vi "oa_SCL Draw Grid.vi"(8 "grid cosmetics":T1={"line color"=39168, "text color"=65280, "tick length"=3, "crossing axes"=FALSE, "visible grid?"=TRUE}, 9 "y scale specs":cluster{"coordinate":i16, "label":string}[](array[cluster]), 10 "x scale specs":cluster{"coordinate":i16, "label":string}[](array[cluster]), 11 "picture":picture) -> (3 "new picture":picture)   [LabVIEW 2017]
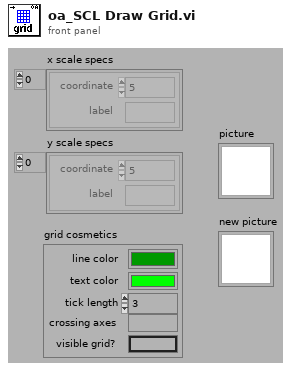
[diagram p1: front panel]
types:
  T1 = cluster{"line color":u32, "text color":u32, "tick length":i16, "crossing axes":bool, "visible grid?":bool}
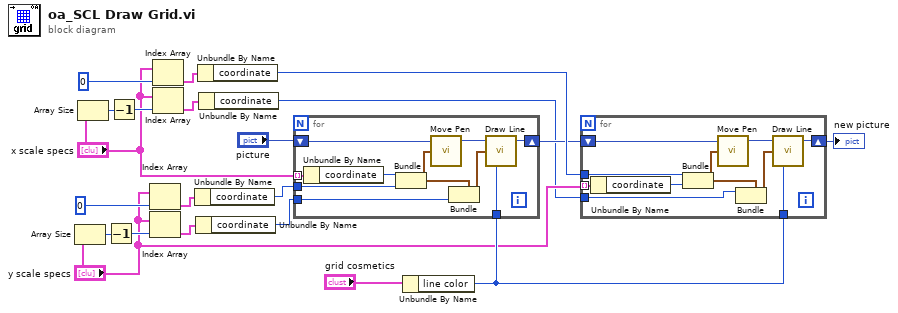
[diagram p0: block diagram]
diagram:
  n1 = Array Size(array="y scale specs") -> (size(s)=w18:i32)
  n2 = Array Size(array="x scale specs") -> (size(s)=w5:i32)
  n3 = Decrement(x=w18) -> (x-1=w19:i32)
  n4 = Decrement(x=w5) -> (x-1=w4:i32)
  n5 = Index Array(array="y scale specs", index=0) -> (element=w16:cluster{"coordinate":i16, "label":string})
  n6 = Index Array(array="y scale specs", index=w19) -> (element=w15:cluster{"coordinate":i16, "label":string})
  n7 = Index Array(array="x scale specs", index=0) -> (element=w7:cluster{"coordinate":i16, "label":string})
  n8 = Index Array(array="x scale specs", index=w4) -> (element=w8:cluster{"coordinate":i16, "label":string})
  n9 = Unbundle By Name(w16) -> ("coordinate"=w14:i16)
  n10 = Unbundle By Name(w15) -> ("coordinate"=w13:i16)
  n11 = Unbundle By Name(w7) -> ("coordinate"=w21:i16)
  n12 = Unbundle By Name(w8) -> ("coordinate"=w1:i16)
  n13 = Unbundle By Name("grid cosmetics") -> ("line color"=w20:u32)
  n14 = for {
    tunnel: "x scale specs" -> [w28] mode=indexing
    tunnel: w14 -> [w26]
    tunnel: w13 -> [w24]
    shift-right: [w31] -> w10
    shift-left: "picture" -> [w29]
    tunnel: w20 -> [w22]
    n15 = Unbundle By Name(w28) -> ("coordinate"=w27:i16)
    n16 = Bundle("coordinate"=w27, "coordinate"=w26) -> (w25:cluster{"coordinate":i16, "coordinate":i16})  [unwired: 1 in]
    n17 = call <vilib>:"Move Pen.vi"("new position"=w25, "picture"=w29) -> ("new picture"=w30:picture)  [unwired: 3 in]
    n18 = Bundle(cluster=w25, "coordinate"=w24) -> (w23:cluster{"coordinate":i16, "coordinate":i16})  [unwired: 1 in]
    n19 = call <vilib>:"Draw Line.vi"("picture"=w30, "end point"=w23, "color(black)"=w22) -> ("new picture"=w31:picture)  [unwired: 6 in]
  }
  n20 = for {
    tunnel: "y scale specs" -> [w38] mode=indexing
    tunnel: w21 -> [w33]
    shift-right: [w41] -> w2
    shift-left: w10 -> [w39]
    tunnel: w20 -> [w35]
    tunnel: w1 -> [w32]
    n21 = Unbundle By Name(w38) -> ("coordinate"=w34:i16)
    n22 = Bundle("coordinate"=w33, "coordinate"=w34) -> (w37:cluster{"coordinate":i16, "coordinate":i16})  [unwired: 1 in]
    n23 = call <vilib>:"Move Pen.vi"("new position"=w37, "picture"=w39) -> ("new picture"=w40:picture)  [unwired: 3 in]
    n24 = Bundle(cluster=w37, "coordinate"=w32) -> (w36:cluster{"coordinate":i16, "coordinate":i16})  [unwired: 1 in]
    n25 = call <vilib>:"Draw Line.vi"("picture"=w40, "end point"=w36, "color(black)"=w35) -> ("new picture"=w41:picture)  [unwired: 6 in]
  }
  "new picture" <- w2
